vi "Read Update Rate (4Hz-100Hz).vi"(8 "error in (no error)":errorcluster, 11 "navX - Base in":refnum<class "navX - Base.lvclass">) -> (0 "error out":errorcluster, 2 "Update Rate (4Hz-100Hz)":u8=4 min=4 max=100 step=1, 3 "navX - Base out":refnum<class "navX - Base.lvclass">)   [LabVIEW 2015, in "navX Library v3.lvlib" / "navX - Base.lvclass"]
uses:
  navX - Base.lvclass
  navX - Base.lvclass/navX - Base.ctl
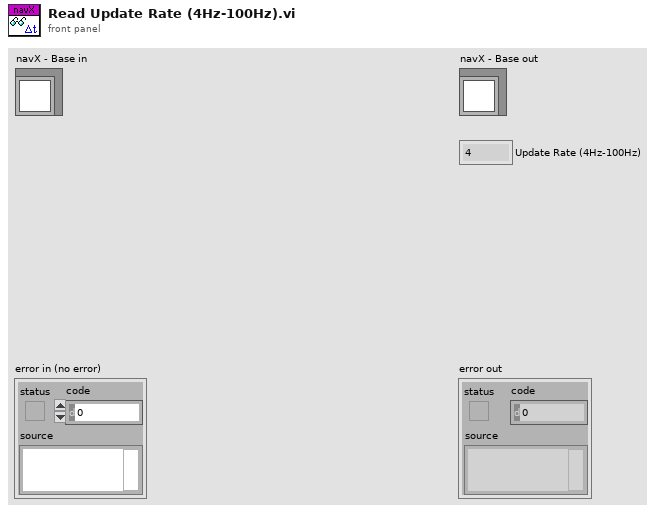
[diagram p1: front panel]
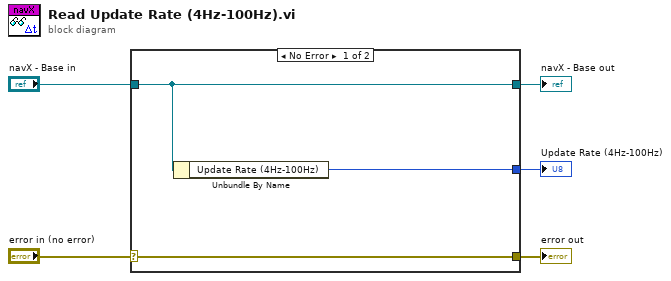
[diagram p0: block diagram]
diagram:
  n1 = case shown="No Error" "error in (no error)" {
    selector: "error in (no error)" -> [w8 w9]
    tunnel: [w8 w9] -> w4
    tunnel: [w7 w10] -> w2
    tunnel: "navX - Base in" -> [w7 w10]
    tunnel: [w6 _] -> w1
    frame No Error {
      n2 = Unbundle By Name(w7) -> ("Update Rate (4Hz-100Hz)"=w6:u8)
    }
    frame Error {
    }
  }
  "error out" <- w4
  "navX - Base out" <- w2
  "Update Rate (4Hz-100Hz)" <- w1
